vi "NI VeriStand - Highlight Node in System Explorer.vi"(8 "error in (no error)":errorcluster, 11 "Item Ref in":T1=18446744073709551615 format="%.0x") -> (0 "error out":errorcluster, 3 "Node Ptr dup":T1=18446744073709551615 format="%.0x")   [LabVIEW 2020, in "Custom Device Utility Library.lvlib"]
doc: "Highlights a custom device item in the <B>System Explorer</B> window configuration tree."
uses:
  <vilib>/NI VeriStand/Custom Device Tools/Custom Device Utility Library/Custom Device Utility Library.lvlib
  <vilib>/NI VeriStand/Custom Device API/Custom Device Item Ref.ctl
  <vilib>/NI VeriStand/Custom Device API/Custom Device API.lvlib
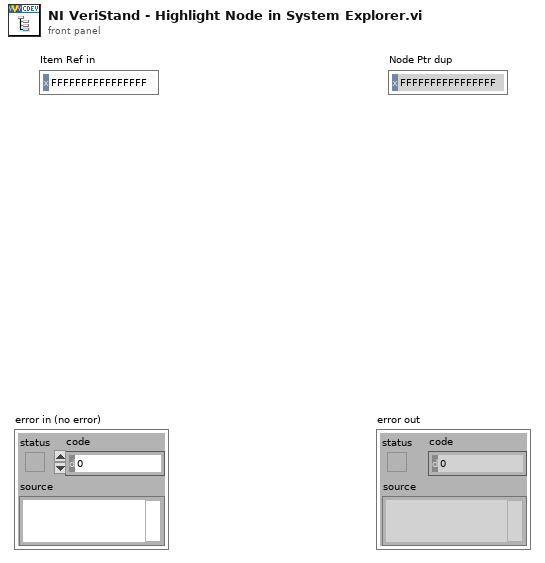
[diagram p1: front panel]
types:
  T1 = typedef "Custom Device API.lvlib/Custom Device Item Ref.ctl" = u64
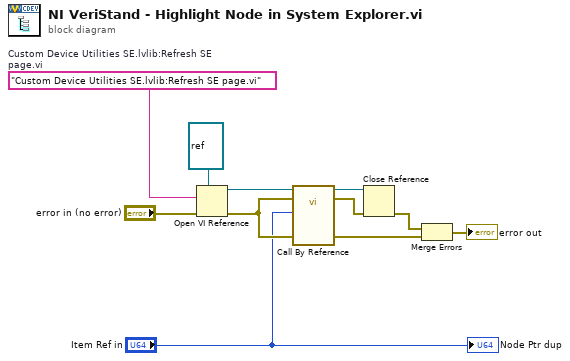
[diagram p0: block diagram]
diagram:
  w11 = "Custom Device Utilities SE.lvlib:Refresh SE page.vi"  # Custom Device Utilities SE.lvlib:Refresh SE page.vi
  n1 = Open VI Reference(type specifier VI Refnum (for type only)=refnum<vi> refnum, vi path=w11, error in (no error)="error in (no error)") -> (vi reference=w4:refnum<vi>, error out=w5:errorcluster)  [unwired: 3 out]
  n2 = call-by-ref "?"(reference=w4, error in=w5, 8:"error in (no error)"=w5, "Node Ptr"="Item Ref in") -> (reference out=w8:refnum<vi>, error out=w9:errorcluster, 0:"error out"=w10:errorcluster)  [unwired: 9 in]
  n3 = Close Reference(reference=w8, error in (no error)=w9) -> (error out=w7:errorcluster)
  n4 = Merge Errors(w7, w10) -> (→"error out":errorcluster)
  "Node Ptr dup" <- "Item Ref in"
